vi "Quaternion_New.vi"(8 "Z":dbl, 9 "Y":dbl, 10 "X":dbl, 11 "W":dbl=1.0) -> (3 "out Quaternion":T1={"R"=1.0, "V"=[0.0, 0.0, 0.0]})   [LabVIEW 2019, in "Trajectory_Library.lvlib"]
doc: "Convenience constructors that takes in x and y values directly instead of having to construct a Translation2d.\n\nParameters:\n - X- The x component of the translational component of the pose.\n - Y - The y component of the translational component of the pose.\n - Rotation (Heading) - The rotational component of the pose.\n\nReturns:\n - OUT POSE - Output POSE"
uses:
  Trajectory_Library.lvlib
  QUATERNION.ctl
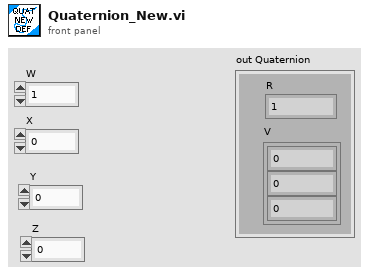
[diagram p1: front panel]
types:
  T1 = typedef "Trajectory_Library.lvlib/QUATERNION.ctl" = cluster{"R":dbl, "V":dbl[]}
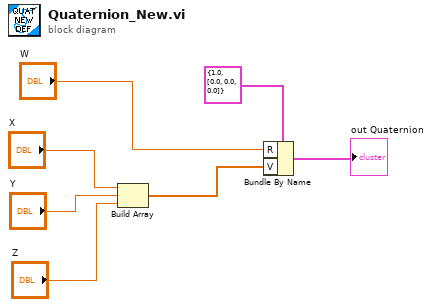
[diagram p0: block diagram]
diagram:
  n1 = Build Array("X", "Y", "Z") -> (w1:dbl[])
  n2 = Bundle By Name(cluster=T1 {"R"=1.0, "V"=[0.0, 0.0, 0.0]} ("sumPOSE"), "R"="W", "V"=w1) -> (→"out Quaternion":T1)
